vi "CM_DetectPulses.vi"(8 "Error In":errorcluster, 11 "Data":dbl[][](array[numeric])) -> (0 "Error out":errorcluster)   [LabVIEW 2016]
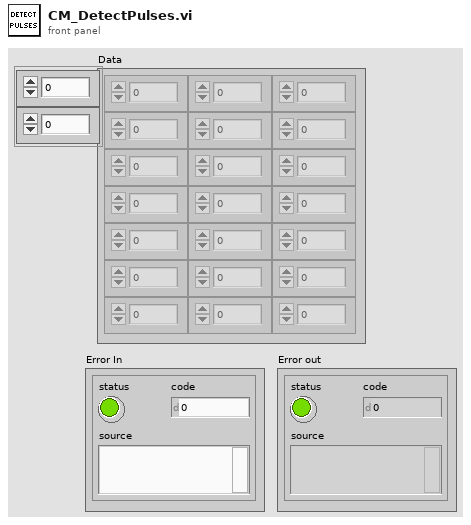
[diagram p1: front panel]
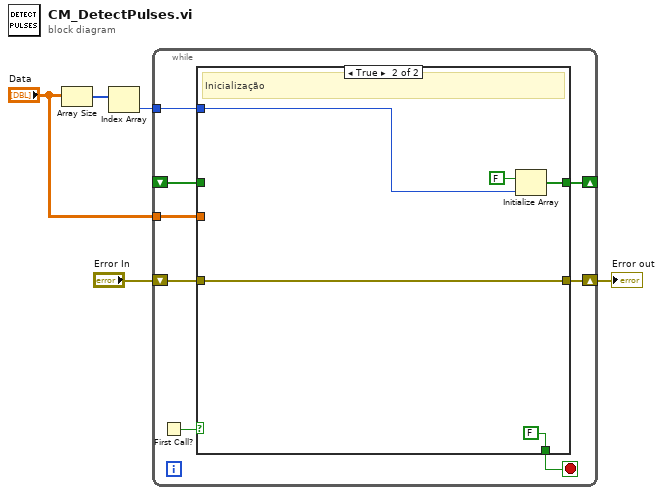
[diagram p0: block diagram]
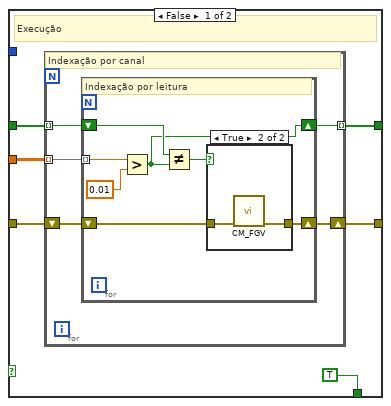
[diagram p2: hidden frame]
diagram:
  n1 = Array Size(array="Data") -> (size(s)=w5:i32[])
  n2 = Index Array(array=w5) -> (element=w4:i32)  [unwired: 1 in]
  n3 = while {
    tunnel: w4 -> [w12]
    shift-right: [w11] -> _
    shift-left: _ -> [w10]
    tunnel: "Data" -> [w9]
    shift-right: [w8] -> w1
    shift-left: "Error In" -> [w7]
    stop <- w13 stop-if-true
    n4 = First Call?() -> (First Call?: T/F=w6:bool)
    n5 = case shown="True" w6 {
      tunnel: [TRUE FALSE] -> w13
      tunnel: w12 -> [_ w38]
      tunnel: [w14 w36] -> w11
      tunnel: w10 -> [w18 _]
      tunnel: w9 -> [w17 _]
      tunnel: [w16 w35] -> w8
      tunnel: w7 -> [w15 w35]
      frame False {
        # "Execução"
        n6 = for {
          tunnel: w18 -> [w24] mode=indexing
          tunnel: w17 -> [w23] mode=indexing
          shift-right: [w22] -> w16
          shift-left: w15 -> [w21]
          tunnel: [w20] -> w14 mode=indexing
          # "Indexação por canal"
          n7 = for {
            shift-right: [w28] -> w20
            shift-left: w24 -> [w29]
            tunnel: w23 -> [w31] mode=indexing
            shift-right: [w26] -> w22
            shift-left: w21 -> [w25]
            # "Indexação por leitura"
            n8 = Greater?(x=w31, y=0.01) -> (0:w28:bool)
            n9 = Not Equal?(x=w29, y=w28) -> (x != y?=w27:bool)
            n10 = case shown="True" w27 {
              tunnel: [w32 w34] -> w26
              tunnel: w25 -> [w32 w33]
              frame False {
              }
              frame True {
                n11 = call "CM_FGV.vi"("Error In"=w33) -> ("Error Out"=w34:errorcluster)  [unwired: 9 in, 1 out]
              }
            }
          }
        }
      }
      frame True {
        # "Inicialização"
        n12 = Initialize Array(FALSE, w38) -> (w36:bool[])
      }
    }
  }
  "Error out" <- w1
